vi "Read Cofiguration.vi"(8 "Error In":errorcluster, 11 "Array":refnum<vi>[](array[refnum])) -> (0 "Error Out":errorcluster)   [LabVIEW 2015]
uses:
  <vilib>/Utility/config.llb/NI_LVConfig.lvlib
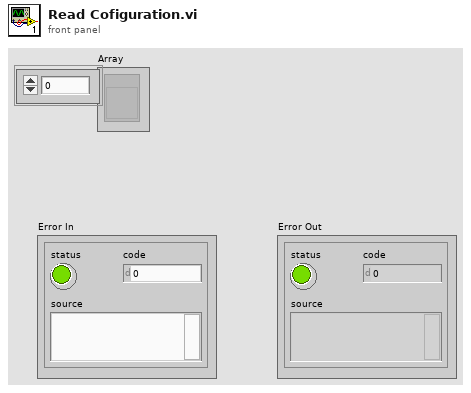
[diagram p1: front panel]
types:
  T1 = typedef "NI_LVConfig.lvlib/Config Data RefNum.ctl" = refnum<k1>
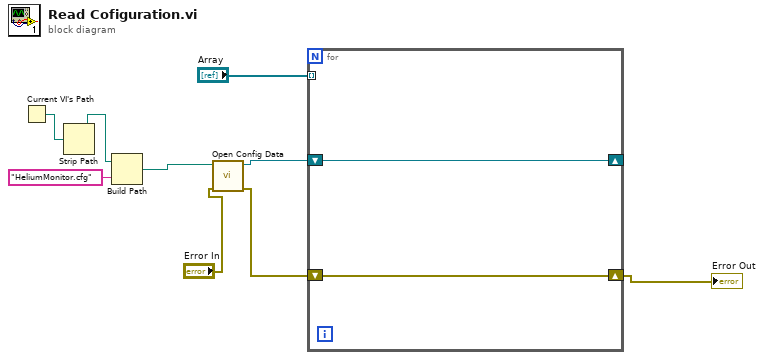
[diagram p0: block diagram]
diagram:
  n1 = Current VI's Path() -> (path=w9:path)
  n2 = Strip Path(path=w9) -> (stripped path=w8:path)  [unwired: 1 out]
  n3 = Build Path(base path=w8, name or relative path="HeliumMonitor.cfg") -> (appended path=w6:path)
  n4 = call <vilib>:"Open Config Data.vi"("error in (no error)"="Error In", "configuration file path"=w6) -> ("error out"=w1:errorcluster, "refnum"=w4:T1)  [unwired: 7 in, 1 out]
  n5 = for {
    tunnel: "Array" -> [_] mode=indexing
    shift-right: [w10] -> _
    shift-left: w4 -> [w10]
    shift-right: [w11] -> w3
    shift-left: w1 -> [w11]
  }
  "Error Out" <- w3
